vi "Fit Circle - 2D Test.vi"() -> ()   [LabVIEW 2023]
uses:
  Vec3d Class/Vec3d.lvclass
panel:
  in  "noise":dbl=0.1 format="%#_13g"
  out "Residual":dbl
  out "error out":errorcluster
  out "Radius":dbl
  out "Center":cluster{"X":dbl, "Y":dbl, "Z":dbl}
  in  "R":dbl=4.0
  in  "Y":dbl=3.0
  in  "X":dbl=2.0
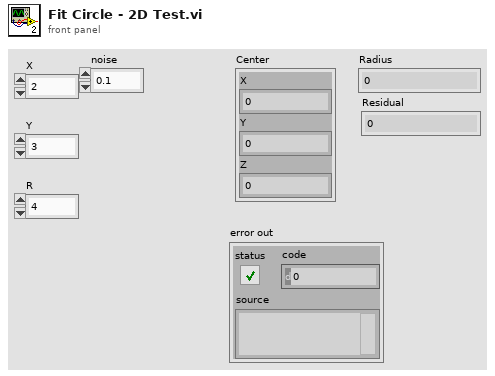
[diagram p1: front panel]
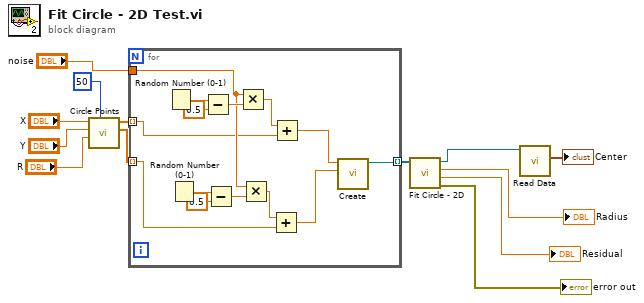
[diagram p0: block diagram]
diagram:
  n1 = call "Circle Points.vi"("N"=50, "Radius"="R", "Y"="Y", "X"="X") -> ("Ys"=w1:dbl[], "Xs"=w2:dbl[])  [unwired: 6 in]
  n2 = for {
    tunnel: [w19] -> w13 mode=indexing
    tunnel: "noise" -> [w18]
    tunnel: w2 -> [w17] mode=indexing
    tunnel: w1 -> [w16] mode=indexing
    n3 = Random Number (0-1)() -> (number: 0 to 1=w27:dbl)
    n4 = Random Number (0-1)() -> (number: 0 to 1=w23:dbl)
    n5 = Subtract(x=w27, y=0.5) -> (x-y=w25:dbl)
    n6 = Subtract(x=w23, y=0.5) -> (x-y=w21:dbl)
    n7 = Multiply(x=w18, y=w25) -> (x*y=w24:dbl)
    n8 = Multiply(x=w18, y=w21) -> (x*y=w20:dbl)
    n9 = Add(x=w20, y=w16) -> (x+y=w14:dbl)
    n10 = Add(x=w24, y=w17) -> (x+y=w15:dbl)
    n11 = call "Create.vi"("Y"=w14, "X"=w15) -> ("Vec3d Class out"=w19:refnum<class "Vec3d.lvclass">)  [unwired: 8 in, 1 out]
  }
  n12 = call "Fit Circle - 2D.vi"("Points"=w13) -> ("error out"=→"error out":errorcluster, "Residual"=→"Residual":dbl, "Radius"=→"Radius":dbl, "Center"=w12:refnum<class "Vec3d.lvclass">)  [unwired: 7 in]
  n13 = call-dynamic "Read Data.vi"("Vec3d Class in"=w12) -> ("Data"=→"Center":cluster{"X":dbl, "Y":dbl, "Z":dbl})  [unwired: 8 in, 2 out]
